vi "Register Keyboard Events.vi"(8 "error in (no error)":errorcluster, 11 "PictureRef":refnum<vi>) -> (0 "error out":errorcluster, 1 "CB VIs":refnum<vi>[](array[refnum]), 2 "event callback refnum":refnum<k27>, 3 "Cluster":T1)   [LabVIEW 2015, in "LV Image Editor Framework.lvlib" / "Image Editor Handler.lvclass"]
uses:
  Image Editor Handler.lvclass
  <vilib>/event_ctls.llb/eventvkey.ctl
  Callbacks/Handler UI Callbacks.lvlib
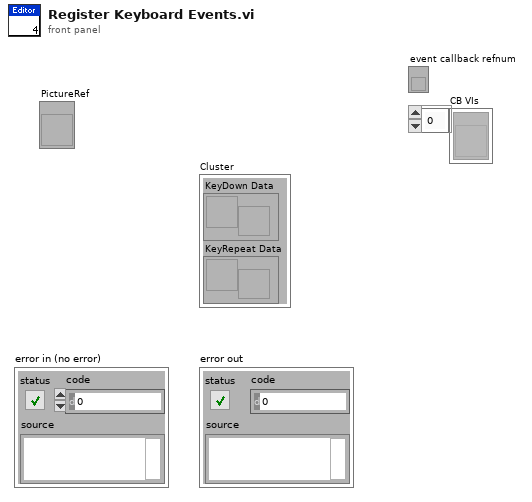
[diagram p1: front panel]
types:
  T1 = cluster{"KeyDown Data":refnum<user-event>, "KeyRepeat Data":refnum<user-event>}
  T2 = typedef "eventvkey.ctl" = enum16{"ASCII", "Enter", "Return", "Shift", "Ctrl", "Alt", "Cmd", "Opt", "Caps", "NumLock", "Clear", "Break", "Up", "Down", "Left", "Right", "Insert", "Delete", "Home", "End", "PageUp", "PageDown", "Escape", "Help", "Pause", "ScrollLock", "F1", "F2", "F3", "F4", "F5", "F6", "F7", "F8", "F9", "F10", "F11", "F12", "F13", "F14", "F15", "F16", "F17", "F18", "F19", "F20", "F21", "F22", "F23", "F24", "Play", "VolumeUp", "VolumeDown", "Mute", "Two Byte Char"}
  T3 = cluster{"Char":i16, "VKey":T2, "ScanCode":i16, "Mods":cluster{"Num Pad":bool, "Menu Key":bool}, "PlatMods":cluster{"Shift":bool, "Ctrl":bool, "Alt":bool, "Cmd":bool, "Opt":bool}, "FocusObj":refnum<vi>}
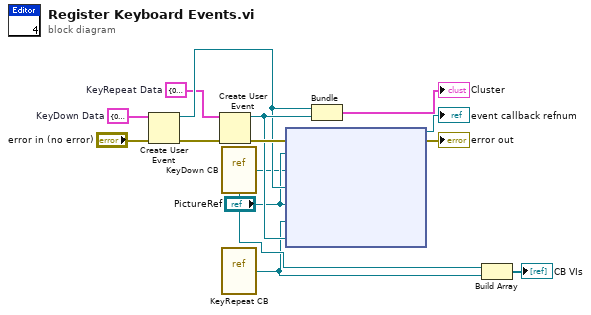
[diagram p0: block diagram]
diagram:
  w7 = T3 {"Char"=0, "VKey"=enum."ASCII", "ScanCode"=0, "Mods"={"Num Pad"=FALSE, "Menu Key"=FALSE}, "PlatMods"={"Shift"=FALSE, "Ctrl"=FALSE, "Alt"=FALSE, "Cmd"=FALSE, "Opt"=FALSE}, "FocusObj"=refnum}  # KeyRepeat Data
  w6 = T3 {"Char"=0, "VKey"=enum."ASCII", "ScanCode"=0, "Mods"={"Num Pad"=FALSE, "Menu Key"=FALSE}, "PlatMods"={"Shift"=FALSE, "Ctrl"=FALSE, "Alt"=FALSE, "Cmd"=FALSE, "Opt"=FALSE}, "FocusObj"=refnum}  # KeyDown Data
  n1 = Create User Event(user event datatype=w6, error in="error in (no error)") -> (user event=w8:refnum<user-event>, error out=w11:errorcluster)
  n2 = Create User Event(user event datatype=w7, error in=w11) -> (user event=w9:refnum<user-event>, error out=w12:errorcluster)
  n3 = vi-ref "KeyDown CB.vi"() -> ("vi reference"=w3:refnum<vi>)
  n4 = vi-ref "KeyRepeat CB.vi"() -> ("vi reference"=w2:refnum<vi>)
  n5 = node(w12, "PictureRef", w3, w8, "PictureRef", w2, w9) -> (→"event callback refnum":refnum<k27>, →"error out":errorcluster)  [unwired: 1 in]
  n6 = Bundle("KeyDown Data"=w8, "KeyRepeat Data"=w9) -> (→"Cluster":T1)  [unwired: 1 in]
  n7 = Build Array(w3, w2) -> (→"CB VIs":refnum<vi>[])
